vi "temptemp.vi"() -> ()   [LabVIEW 2013]
panel:
  out "status":errorcluster
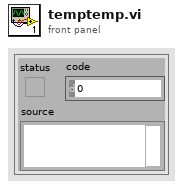
[diagram p1: front panel]
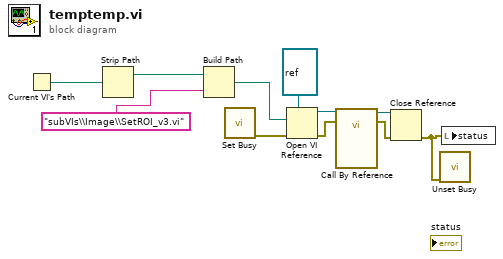
[diagram p0: block diagram]
diagram:
  n1 = Current VI's Path() -> (path=w10:path)
  n2 = Strip Path(path=w10) -> (stripped path=w11:path)  [unwired: 1 out]
  n3 = Build Path(base path=w11, name or relative path="subVIs\\Image\\SetROI_v3.vi") -> (appended path=w9:path)
  n4 = call <vilib>:"Set Busy.vi"() -> ("error out"=w7:errorcluster)  [unwired: 10 in, 1 out]
  n5 = Open VI Reference(type specifier VI Refnum (for type only)=refnum<vi> refnum, vi path=w9, error in (no error)=w7) -> (vi reference=w5:refnum<vi>, error out=w3:errorcluster)  [unwired: 3 in]
  n6 = call-by-ref "?"(reference=w5, error in=w3) -> (reference out=w4:refnum<vi>, error out=w2:errorcluster)  [unwired: 1 in]
  n7 = Close Reference(reference=w4, error in (no error)=w2) -> (error out=w6:errorcluster)
  n8 = call <vilib>:"Unset Busy.vi"("error in (no error)"=w6) -> ()  [unwired: 10 in, 1 out]
  n9 = local write "status"(w6) -> ()
